vi "TakeImages.vi"() -> ()   [LabVIEW 2019]
uses:
  <vilib>/userDefined/High Color/IMAQdx.ctl
  <vilib>/vision/driver/NI_Vision_Acquisition_Software.lvlib
panel:
  in  "ImageVsPosition":path=path "C:/Users/TTUHEP/Pictures/SensorPics/ImageVsPosition.txt"
  in  "Operation":enum16{"ImageTaker", "VacuumControl"}(ring)
  out "NyCurrent":i32
  out "NxCurrent":i32
  out "NyTotal":i32
  out "NxTotal":i32
  out "Error Out":errorcluster
  out "ImageVsPosition":string
  in  "OutputDirectory":string="C:\\Users\\TTUHEP\\Pictures\\SensorPics\\"
  in  "AbortAutoFocus":bool
  in  "AutoFocus":bool
  in  "SafeMaxZ":dbl=77.0 format="%#_13g"
  out "Image":T1(plugin-control)
  in  "RectY":dbl=76.399
  in  "RectX":dbl=167.899
  in  "CenterZ":dbl=75.331
  in  "CenterY":dbl=1006.197
  in  "CenterX":dbl=844.118
  out "VacState1":T2
  out "DecimalExpected":u32
  out "DecimalOut":u32
  in  "ControlType":T3(ring)
  in  "Zone":enum16{"ZoneA", "ZoneB", "ZoneC", "ZoneD"}(ring)
  in  "Position":enum16{"1", "2"}(ring)
  in  "Error In":errorcluster
  in  "DecimalIn":u8
  in  "Switches":T4
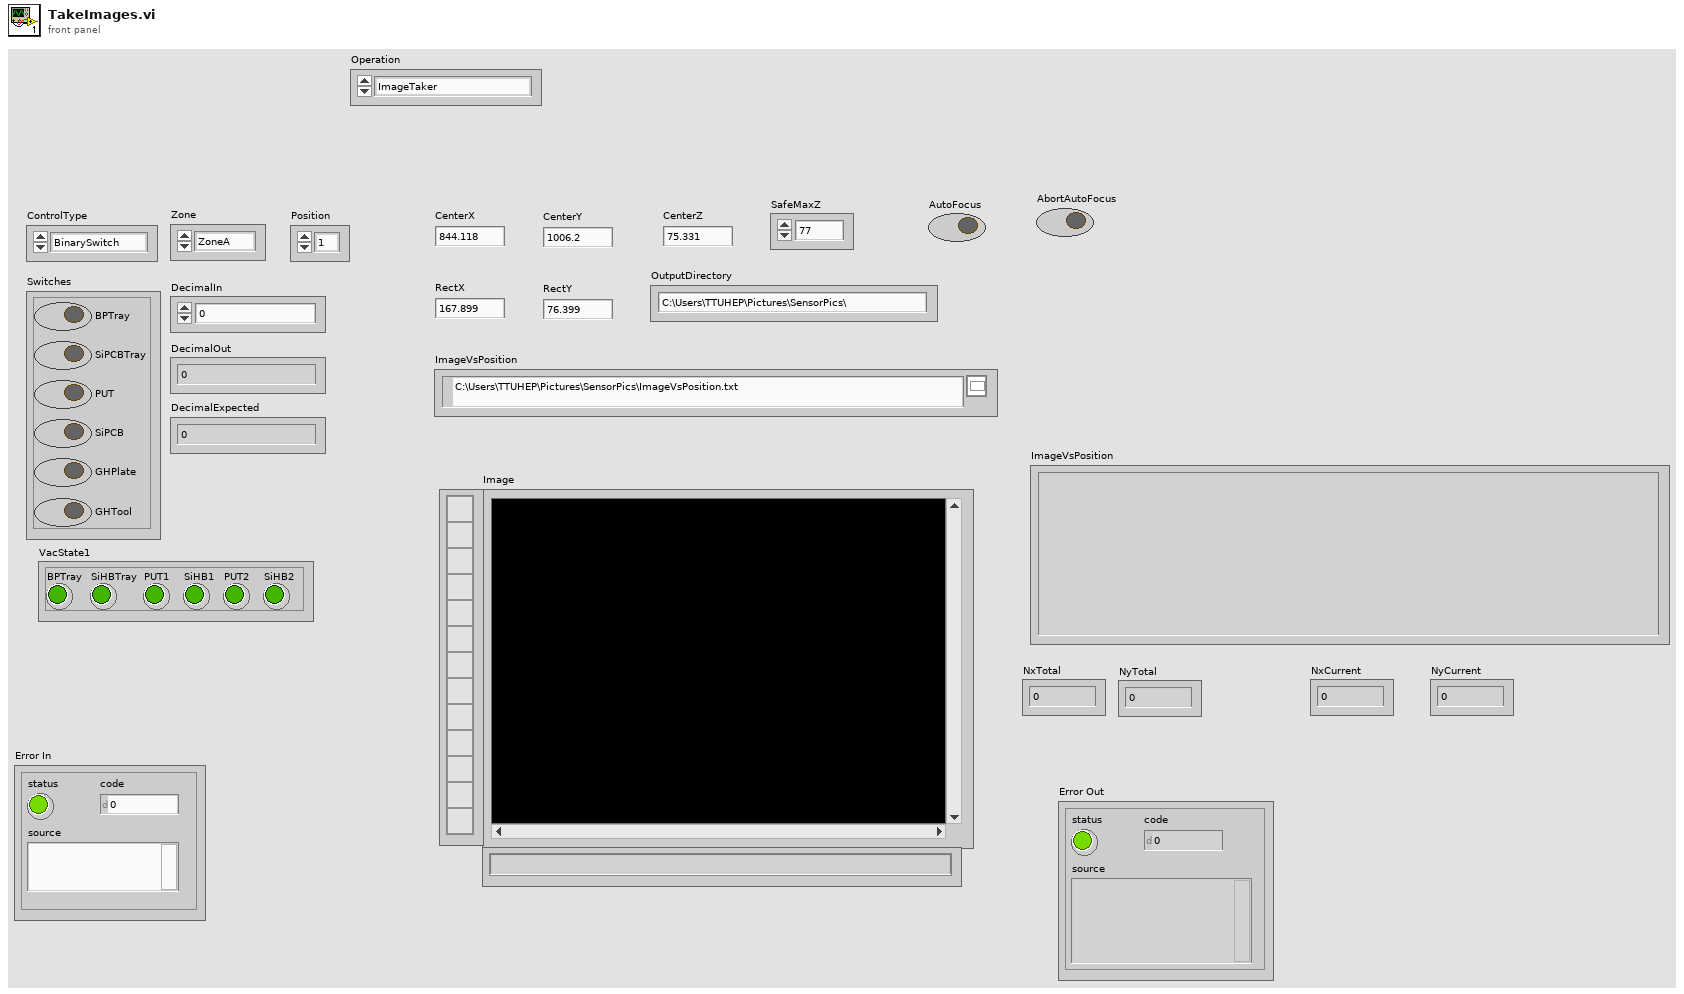
[diagram p1: front panel]
types:
  T1 = typedef "IMAQ Image.ctl" = refnum<image>
  T2 = cluster{"BPTray":bool, "SiHBTray":bool, "PUT1":bool, "SiHB1":bool, "PUT2":bool, "SiHB2":bool, "NC":bool, "NC":bool, "NC":bool}
  T3 = enum16{"BinarySwitch", "DecimalSwitch", "Conversion"}
  T4 = cluster{"BPTray":bool, "SiPCBTray":bool, "PUT":bool, "SiPCB":bool, "GHPlate":bool, "GHTool":bool}
  T5 = typedef "IMAQdx.ctl" = refnum<k21>
  T6 = enum16{"open", "replace", "create", "open or create", "replace or create", "replace or create with confirmation"}
  T7 = typedef "Image Type" = u32
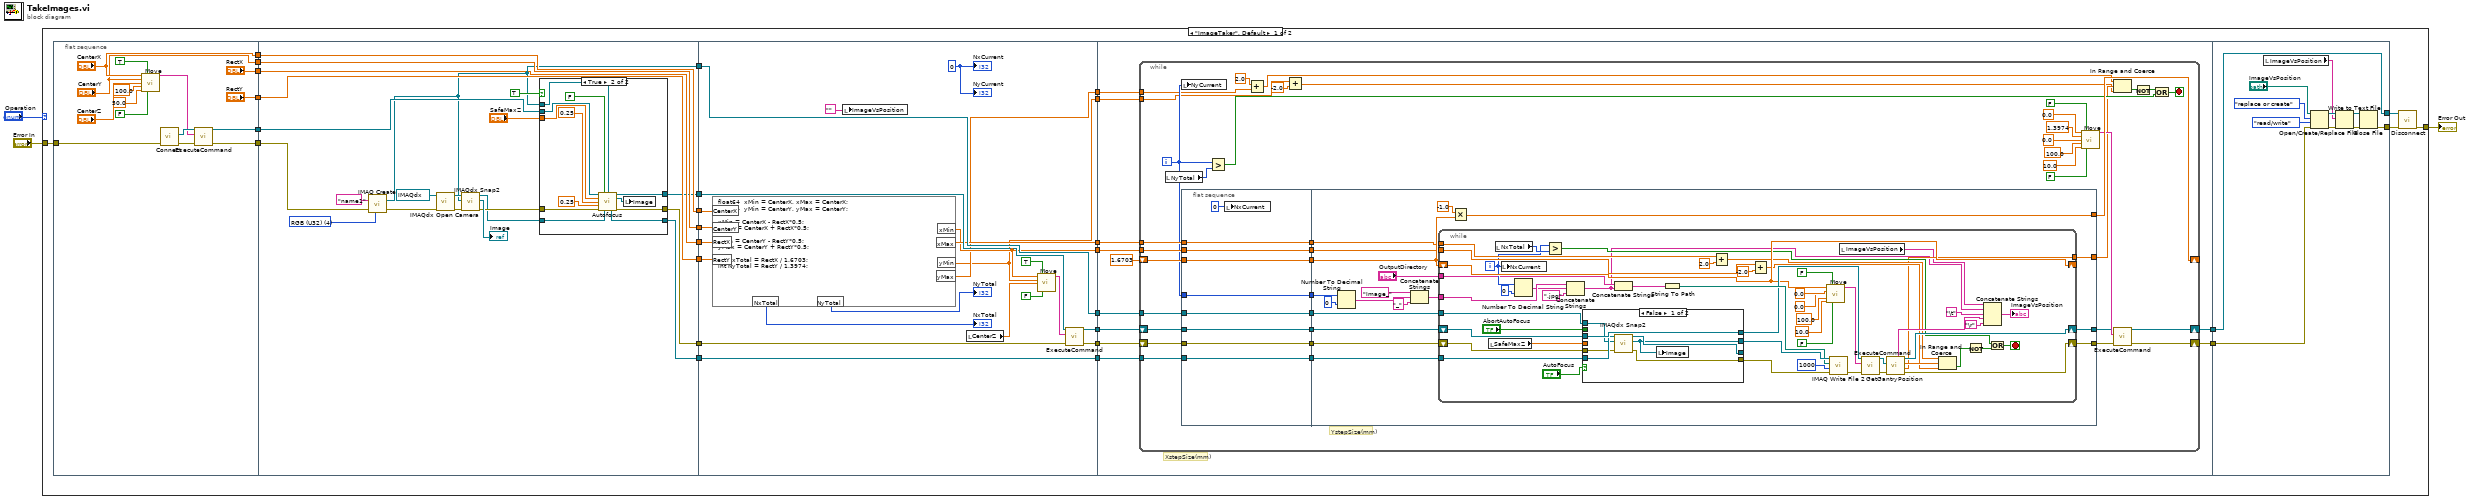
[diagram p0: block diagram]
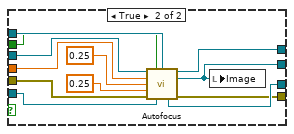
[diagram p3: hidden frame]
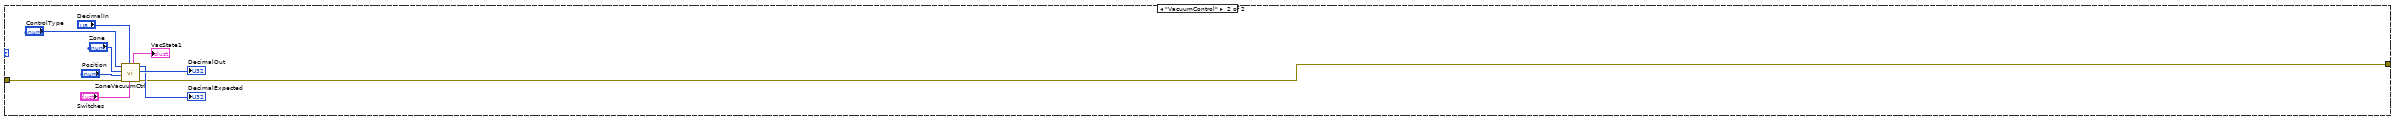
[diagram p4: hidden frame]
diagram:
  n1 = case shown="\"ImageTaker\", Default" "Operation" {
    tunnel: [w8 w266] -> w1
    tunnel: "Error In" -> [w6 w267]
    frame "ImageTaker", Default {
      n2 = flat-sequence {
        tunnel: [w44] -> w31
        tunnel: [w43] -> w30
        tunnel: ["RectX"] -> w29
        tunnel: ["RectY"] -> w28
        tunnel: ["CenterX"] -> w27
        tunnel: ["CenterY"] -> w26
        tunnel: w6 -> [w32]
        tunnel: w31 -> [w55]
        tunnel: [w51] -> w25
        tunnel: w30 -> [w57]
        tunnel: [w50] -> w24
        tunnel: w29 -> [w67]
        tunnel: [w67] -> w23
        tunnel: w28 -> [w66]
        tunnel: [w66] -> w22
        tunnel: w27 -> [w65]
        tunnel: [w65] -> w21
        tunnel: w26 -> [w64]
        tunnel: [w64] -> w20
        tunnel: [w49] -> w19
        tunnel: [w47] -> w18
        tunnel: w25 -> [w95]
        tunnel: w24 -> [w97]
        tunnel: w23 -> [w101]
        tunnel: w22 -> [w100]
        tunnel: w21 -> [w99]
        tunnel: w20 -> [w98]
        tunnel: w19 -> [w94]
        tunnel: [w94] -> w17
        tunnel: [w93] -> w16
        tunnel: [w92] -> w15
        tunnel: w18 -> [w91]
        tunnel: [w91] -> w14
        tunnel: [w90] -> w13
        tunnel: [w89] -> w12
        tunnel: [w85] -> w11
        tunnel: [w84] -> w10
        tunnel: w17 -> [w115]
        tunnel: w16 -> [w114]
        tunnel: w15 -> [w113]
        tunnel: w14 -> [w112]
        tunnel: w13 -> [w110]
        tunnel: w12 -> [w109]
        tunnel: w11 -> [w108]
        tunnel: w10 -> [w107]
        tunnel: [w105] -> w5
        tunnel: [w106] -> w4
        tunnel: [w265] -> w7
        tunnel: [w256] -> w9
        tunnel: w5 -> [w265]
        tunnel: w4 -> [w259]
        frame #0 {
          n3 = call "Move.vi"("X"="CenterX", "Absolute"=TRUE, "Y"="CenterY", "Z"="CenterZ", "SpeedXY (mm/s)"=100.0, "SpeedZ (mm/s)"=50.0, "Move Z first"=FALSE) -> ("Position Gcode"=w37:string)  [unwired: 8 in]
          n4 = call "Connect.vi"("error in (no error)"=w32) -> ("error out"=w45:errorcluster, "controller"=w46:refnum<k24>)  [unwired: 9 in]
          n5 = call "ExecuteCommand.vi"("error in (no error)"=w45, "Command Code"=w37, "controller in"=w46) -> ("error out"=w43:errorcluster, "controller out"=w44:refnum<k24>)  [unwired: 6 in, 1 out]
        }
        frame #1 {
          w60 = T7 4 items=["Grayscale (U8)", "Grayscale (I16)", "Grayscale (SGL)", "Complex (CSG)", "RGB (U32)", "HSL (U32)", "RGB (U64)", "Grayscale (U16)"] ("Image Type")
          n6 = call "IMAQ Create"("Image Name"="name1" ("ImageName"), "Image Type"=w60, "error in (no error)"=w57) -> ("New Image"=w47:T1, "error out"=w62:errorcluster)  [unwired: 2 in]
          n7 = call <vilib>:"IMAQdx Open Camera.vi"("error in"=w62, "Session In"=T5 "cam1" ("Camera")) -> ("error out"=w58:errorcluster, "Session Out"=w59:T5)  [unwired: 8 in]
          n8 = call <vilib>:"IMAQdx Snap2.vi"("error in"=w58, "Image In"=w47, "Session In"=w59) -> ("error out"=w53:errorcluster, "Image Out"=→"Image":T1, "Session Out"=w52:T5)  [unwired: 6 in]
          n9 = case shown="True" TRUE {
            tunnel: w55 -> [w69 w82]
            tunnel: "SafeMaxZ" -> [_ w81]
            tunnel: w53 -> [w68 w78]
            tunnel: w52 -> [w70 w77]
            tunnel: w47 -> [_ w76]
            tunnel: [w69 w75] -> w51
            tunnel: [w70 w73] -> w49
            tunnel: [w68 w72] -> w50
            frame False {
            }
            frame True {
              n10 = call "Autofocus.vi"("controller in"=w82, "AbortAutoFocus"=FALSE, "ImageIn"=w76, "SafeMaxZ"=w81, "InitialStepSize"=0.25, "Tolerance"=0.25, "error in (no error)"=w78, "SessionIn"=w77) -> ("controller out"=w75:refnum<k24>, "Image"=w74:T1, "Session Out"=w73:T5, "error out"=w72:errorcluster)  [unwired: 2 in, 2 out]
              n11 = local write "Image"(w74) -> ()
            }
          }
        }
        frame #2 {
          w86 = 0 ("NxCurrent")
          n12 = formula code="float64  xMin = CenterX, xMax = CenterX;\nfloat64  yMin = CenterY, yMax = CenterY;\n\nxMin = CenterX - RectX*0.5;\nxMax = CenterX + RectX*0.5;\n\nyMin = CenterY - RectY*0.5;\nyMax = CenterY + RectY*0.5;\n\nint NxTotal = RectX / 1.6703;\nint NyTotal = RectY / 1.3974;"("CenterX"=w99, "CenterY"=w98, "RectX"=w101, "RectY"=w100) -> ("xMin"=w89:dbl, "xMax"=w90:dbl, "yMin"=w84:dbl, "yMax"=w85:dbl, "NxTotal"=→"NxTotal":i32, "NyTotal"=→"NyTotal":i32)
          n13 = local write "ImageVsPosition"("") -> ()
          n14 = local read "CenterZ"() -> (w104:dbl)
          n15 = call "Move.vi"("X"=w89, "Absolute"=TRUE, "Y"=w84, "Z"=w104, "Move Z first"=FALSE) -> ("Position Gcode"=w96:string)  [unwired: 10 in]
          n16 = call "ExecuteCommand.vi"("error in (no error)"=w97, "Command Code"=w96, "controller in"=w95) -> ("error out"=w92:errorcluster, "controller out"=w93:refnum<k24>)  [unwired: 6 in, 1 out]
          "NxCurrent" <- w86
          "NyCurrent" <- w86
        }
        frame #3 {
          # "XstepSize(mm)"
          n17 = while {
            tunnel: w115 -> [w156]
            tunnel: w112 -> [w153]
            shift-right: [w151] -> _
            shift-left: 1.6703 -> [w152]
            shift-right: [w144] -> w105
            shift-left: w114 -> [w155]
            shift-right: [w139] -> w106
            shift-left: w113 -> [w154]
            tunnel: w110 -> [w138]
            tunnel: w109 -> [w137]
            tunnel: w108 -> [w122]
            tunnel: w107 -> [w119]
            i -> [w127]
            stop <- w126 stop-if-true
            # "YstepSize(mm)"
            n18 = local read "NyTotal"() -> (w128:i32)
            n19 = local write "NyCurrent"(w127) -> ()
            n20 = flat-sequence {
              tunnel: w137 -> [w158]
              tunnel: w138 -> [w159]
              tunnel: w152 -> [w160]
              tunnel: w127 -> [w161]
              tunnel: w153 -> [w162]
              tunnel: w154 -> [w163]
              tunnel: w155 -> [w164]
              tunnel: w156 -> [w165]
              tunnel: [w165] -> w136
              tunnel: [w164] -> w135
              tunnel: [w163] -> w134
              tunnel: [w162] -> w133
              tunnel: [w161] -> w132
              tunnel: [w160] -> w131
              tunnel: [w159] -> w130
              tunnel: [w158] -> w129
              tunnel: [w172] -> w151
              tunnel: [w171] -> w145
              tunnel: [w170] -> w140
              tunnel: w136 -> [w184]
              tunnel: w135 -> [w183]
              tunnel: w134 -> [w182]
              tunnel: w133 -> [w181]
              tunnel: w132 -> [w180]
              tunnel: w131 -> [w173]
              tunnel: w130 -> [w169]
              tunnel: w129 -> [w168]
              tunnel: [w167] -> w124
              frame #0 {
                n21 = local write "NxCurrent"(0 ("NxCurrent")) -> ()
              }
              frame #1 {
                n22 = Number To Decimal String(number=w180, width (-)=i16 0) -> (decimal integer string=w178:string)
                n23 = Concatenate Strings("Image_" ("string"), w178, "_" ("string")) -> (w175:string)
                n24 = while {
                  tunnel: w184 -> [w233]
                  tunnel: w181 -> [w229]
                  tunnel: w175 -> [w224]
                  shift-right: [w205] -> _
                  shift-left: w173 -> [w205]
                  shift-right: [w209] -> w171
                  shift-left: w183 -> [w232]
                  shift-right: [w208] -> w170
                  shift-left: w182 -> [w230]
                  tunnel: w169 -> [w203]
                  tunnel: w168 -> [w199]
                  tunnel: [w193] -> w167
                  tunnel: "OutputDirectory" -> [w187]
                  i -> [w196]
                  stop <- w194 stop-if-true
                  n25 = local read "SafeMaxZ"() -> (w231:dbl)
                  n26 = local read "NxTotal"() -> (w197:i32)
                  n27 = local write "NxCurrent"(w196) -> ()
                  n28 = Number To Decimal String(number=w196, width (-)=i16 0) -> (decimal integer string=w223:string)
                  n29 = Greater?(x=w196, y=w197) -> (0:w195:bool)
                  n30 = Concatenate Strings(w224, w223, ".jpg" ("string")) -> (w185:string)
                  n31 = case shown="False" "AutoFocus" {
                    tunnel: w232 -> [w242 w254]
                    tunnel: w231 -> [_ w253]
                    tunnel: w230 -> [w239 w250]
                    tunnel: w233 -> [w241 w249]
                    tunnel: w229 -> [w240 w248]
                    tunnel: [w242 w247] -> w214
                    tunnel: [w237 w246] -> _
                    tunnel: [w238 w245] -> w226
                    tunnel: "AbortAutoFocus" -> [_ w244]
                    tunnel: [w236 w243] -> w227
                    frame False {
                      n32 = call <vilib>:"IMAQdx Snap2.vi"("error in"=w239, "Image In"=w240, "Session In"=w241) -> ("error out"=w238:errorcluster, "Image Out"=w236:T1, "Session Out"=w237:T5)  [unwired: 6 in]
                      n33 = local write "Image"(w236) -> ()
                    }
                    frame True {
                      n34 = call "Autofocus.vi"("controller in"=w254, "AbortAutoFocus"=w244, "ImageIn"=w248, "SafeMaxZ"=w253, "InitialStepSize"=0.25, "Tolerance"=0.25, "error in (no error)"=w250, "SessionIn"=w249) -> ("controller out"=w247:refnum<k24>, "Image"=w243:T1, "Session Out"=w246:T5, "error out"=w245:errorcluster)  [unwired: 2 in, 2 out]
                      n35 = local write "Image"(w243) -> ()
                    }
                  }
                  n36 = Concatenate Strings(w187, w185) -> (w186:string)
                  n37 = String To Path(string=w186) -> (path=w221:path)
                  n38 = Add(x=w203, y=2.0) -> (x+y=w201:dbl)
                  n39 = Add(x=w199, y=-2.0) -> (x+y=w200:dbl)
                  n40 = call "Move.vi"("X"=w205, "Absolute"=FALSE, "Y"=0.0, "Z"=0.0, "SpeedXY (mm/s)"=100.0, "SpeedZ (mm/s)"=10.0, "Move Z first"=FALSE) -> ("Position Gcode"=w213:string)  [unwired: 8 in]
                  n41 = call-poly "IMAQ Write File 2"("error in (no error)"=w226, "Image Quality"=u32 1000, "File Path"=w221, "Image"=w227) -> ("error out"=w212:errorcluster)  [unwired: 6 in, 1 out]
                  n42 = local read "ImageVsPosition"() -> (w191:string)
                  n43 = call "ExecuteCommand.vi"("error in (no error)"=w212, "Command Code"=w213, "controller in"=w214) -> ("error out"=w210:errorcluster, "controller out"=w211:refnum<k24>)  [unwired: 6 in, 1 out]
                  n44 = call "GetGantryPosition.vi"("error in (no error)"=w210, "Controller In"=w211) -> ("error out"=w208:errorcluster, "Position Y"=w193:dbl, "Position X"=w204:dbl, "controller out"=w209:refnum<k24>, "Position_XYZ"=w206:string)  [unwired: 3 in, 2 out]
                  n45 = In Range and Coerce(upper limit=w201, x=w204, lower limit=w200) -> (In Range?=w190:bool)  [unwired: 1 out]
                  n46 = Not(x=w190) -> (.not. x?=w189:bool)
                  n47 = Concatenate Strings(w191, w185, "\t", w206, "\r") -> (→"ImageVsPosition":string)
                  n48 = Or(x=w195, y=w189) -> (x .or. y?=w194:bool)
                }
                n49 = Multiply(x=-1.0, y=w173) -> (x*y=w172:dbl)
              }
            }
            n50 = Greater?(x=w127, y=w128) -> (0:w125:bool)
            n51 = Add(x=2.0, y=w122) -> (x+y=w121:dbl)
            n52 = Add(x=w119, y=-2.0) -> (x+y=w120:dbl)
            n53 = call "Move.vi"("X"=0.0 ("Y"), "Absolute"=FALSE, "Y"=1.3974, "Z"=0.0, "SpeedXY (mm/s)"=100.0, "SpeedZ (mm/s)"=10.0, "Move Z first"=FALSE) -> ("Position Gcode"=w146:string)  [unwired: 8 in]
            n54 = In Range and Coerce(upper limit=w121, x=w124, lower limit=w120) -> (In Range?=w117:bool)  [unwired: 1 out]
            n55 = call "ExecuteCommand.vi"("error in (no error)"=w140, "Command Code"=w146, "controller in"=w145) -> ("error out"=w139:errorcluster, "controller out"=w144:refnum<k24>)  [unwired: 6 in, 1 out]
            n56 = Not(x=w117) -> (.not. x?=w116:bool)
            n57 = Or(x=w116, y=w125) -> (x .or. y?=w126:bool)
          }
        }
        frame #4 {
          n58 = local read "ImageVsPosition"() -> (w255:string)
          n59 = Open/Create/Replace File(file path (use dialog)="ImageVsPosition", error in=w259, operation (0:open)=T6."replace or create", access (0:read/write)=enum16{"read/write", "read-only", "write-only"}."read/write") -> (refnum out=w263:refnum<file>, error out=w262:errorcluster)  [unwired: 2 in, 1 out]
          n60 = Write to Text File(file (use dialog)=w263, text=w255, error in=w262) -> (refnum out=w260:refnum<file>, error out=w261:errorcluster)  [unwired: 1 in, 1 out]
          n61 = Close File(refnum=w260, error in=w261) -> (error out=w256:errorcluster)  [unwired: 1 out]
        }
      }
      n62 = call "Disconnect.vi"("error in (no error)"=w9, "controller"=w7) -> ("error out"=w8:errorcluster)  [unwired: 9 in]
    }
    frame "VacuumControl" {
      n63 = call "ZoneVacuumCtrl.vi"("Switches"="Switches", "DecimalIn"="DecimalIn", "Error In"=w267, "Position"="Position", "Zone"="Zone", "ControlType"="ControlType") -> ("Error Out"=w266:errorcluster, "DecimalOut"=→"DecimalOut":u32, "DecimalExpected"=→"DecimalExpected":u32, "VacState1"=→"VacState1":T2)  [unwired: 1 in, 1 out]
    }
  }
  "Error Out" <- w1
